vi "myRIO_BRig_RT_dataTrial_iState.vi"() -> (2 "output_iState":i32)   [LabVIEW 2014]
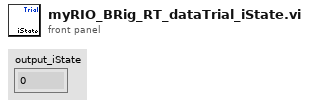
[diagram p1: front panel]
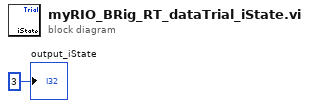
[diagram p0: block diagram]
diagram:
  "output_iState" <- 3 ("output_iBlock")
